vi "Translator.FormatEnumDst.vi"(1 "text in":string) -> (0 "text out":string)   [LabVIEW 2016]
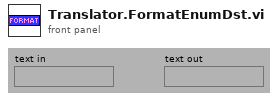
[diagram p1: front panel]
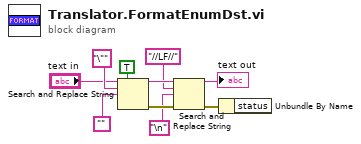
[diagram p0: block diagram]
diagram:
  n1 = Search and Replace String(replace all?=TRUE ("replace all? (F)"), input string="text in", search string="\"", replace string="") -> (result string=w3:string, error out=w4:errorcluster)  [unwired: 4 in, 2 out]
  n2 = Search and Replace String(input string=w3, search string="//LF//", replace string="\n", error in=w4) -> (result string=→"text out":string, error out=w5:errorcluster)  [unwired: 1 in, 5 out]
  n3 = Unbundle By Name(w5) -> ()  [unwired: 1 out]
